vi "Get Table Path.vi"(8 "error in (no error)":errorcluster, 10 "Table Name":string, 11 "Data.PG":refnum<class "LV-Data.PGSQL.lvclass">) -> (0 "error out":errorcluster, 1 "Exists?":bool, 2 "Table Path":string, 3 "Data.PG out":refnum<class "LV-Data.PGSQL.lvclass">)   [LabVIEW 2016, in "LV-Data.PGSQL.lvclass"]
uses:
  LV-Data.PGSQL.lvclass
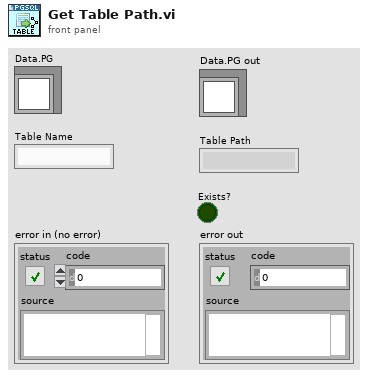
[diagram p1: front panel]
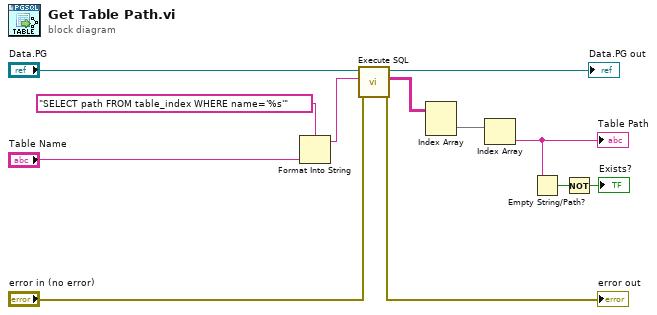
[diagram p0: block diagram]
diagram:
  n1 = Format Into String(format string="SELECT path FROM table_index WHERE name='%s'", "Table Name") -> (resulting string=w10:string)  [unwired: 2 in, 1 out]
  n2 = call "Execute SQL.vi"("error in"="error in (no error)", "SQL"=w10, "LV-Data.PGSQL"="Data.PG") -> ("error out"=→"error out":errorcluster, "Result"=w5:string[][], "LV-Data.PGSQL out"=→"Data.PG out":refnum<class "LV-Data.PGSQL.lvclass">)  [unwired: 6 in]
  n3 = Index Array(array=w5) -> (element=w12:string[])  [unwired: 2 in]
  n4 = Index Array(array=w12) -> (element=w3:string)  [unwired: 1 in]
  "Table Path" <- w3
  n5 = Empty String/Path?(string/path=w3) -> (empty?=w2:bool)
  n6 = Not(x=w2) -> (.not. x?=→"Exists?":bool)
